vi "CheckStatus.vi"(8 "error in":errorcluster, 9 "State":T6, 11 "Hardware Configuration":T1={"Task ID"=0, "Volume"=0.0, "Data"={"SignalType"=enum."SineWave", "WhiteNoiseSettings"={"Generate New Data"=FALSE, "Save"=FALSE, "Filter"=TRUE, "Gain"=0}, "SineWaveSttings"={"Frequency"=0.0, "Amplitude"=0.0}}, "Generated Data"={"t0"=timestamp(0 s since 1904-01-01), "dt"=1.0, "Y"=[]}} {"task ID out" format="%.0x"}) -> (0 "error out":errorcluster, 1 "State":T6, 3 "Hardware Configuration":T1={"Task ID"=0, "Volume"=0.0, "Data"={"SignalType"=enum."SineWave", "WhiteNoiseSettings"={"Generate New Data"=FALSE, "Save"=FALSE, "Filter"=TRUE, "Gain"=0}, "SineWaveSttings"={"Frequency"=0.0, "Amplitude"=0.0}}, "Generated Data"={"t0"=timestamp(0 s since 1904-01-01), "dt"=1.0, "Y"=[]}} {"task ID out" format="%.0x"})   [LabVIEW 2022 SP3]
uses:
  Output Hardware Configuration.ctl
  <vilib>/sound2/lvsound2.llb/Sound Output Task ID.ctl
  Data.ctl
  WhiteNoiseSettings.ctl
  SineWaveSettings.ctl
  Output State.ctl
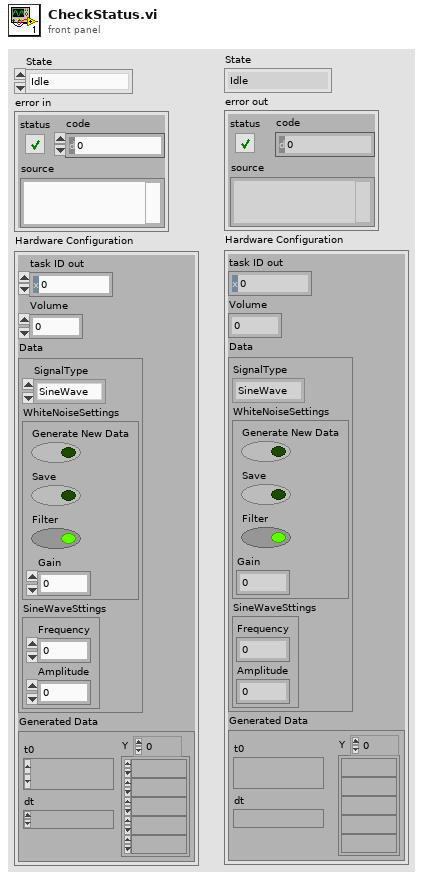
[diagram p1: front panel]
types:
  T1 = typedef "Output Hardware Configuration.ctl" = cluster{"Task ID":T2, "Volume":dbl, "Data":T3, "Generated Data":waveform(dbl)}
  T2 = typedef "Sound Output Task ID.ctl" = u32
  T3 = typedef "Data.ctl" = cluster{"SignalType":enum16{"WhiteNoise", "SineWave"}, "WhiteNoiseSettings":T4, "SineWaveSttings":T5}
  T4 = typedef "WhiteNoiseSettings.ctl" = cluster{"Generate New Data":bool, "Save":bool, "Filter":bool, "Gain":i32}
  T5 = typedef "SineWaveSettings.ctl" = cluster{"Frequency":dbl, "Amplitude":dbl}
  T6 = typedef "Output State.ctl" = enum16{"Idle", "Running"}
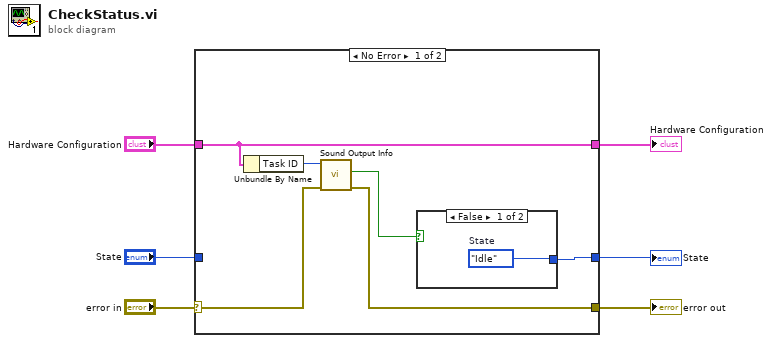
[diagram p0: block diagram]
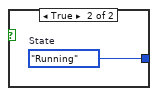
[diagram p2: hidden frame]
diagram:
  n1 = case shown="No Error" "error in" {
    selector: "error in" -> [w11 w17]
    tunnel: [w10 w17] -> w5
    tunnel: "Hardware Configuration" -> [w7 w16]
    tunnel: [w7 w16] -> w3
    tunnel: [w8 w15] -> w2
    tunnel: "State" -> [_ w15]
    frame No Error {
      n2 = Unbundle By Name(w7) -> ("Task ID"=w12:T2)
      n3 = call <vilib>:"Sound Output Info.vi"("error in (no error)"=w11, "task ID"=w12) -> ("error out"=w10:errorcluster, "is playing?"=w9:bool)  [unwired: 6 in, 2 out]
      n4 = case shown="False" w9 {
        tunnel: [w13 w14] -> w8
        frame False {
          w13 = Output_State."Idle"  # State
        }
        frame True {
          w14 = Output_State."Running"  # State
        }
      }
    }
    frame Error {
    }
  }
  "error out" <- w5
  "Hardware Configuration" <- w3
  "State" <- w2
